vi "Tester 1.vi"() -> ()   [LabVIEW 2020]
doc: "211353135"
panel:
  in  "Numeric":i32
  # "Tester 1"
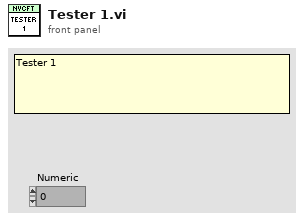
[diagram p1: front panel]
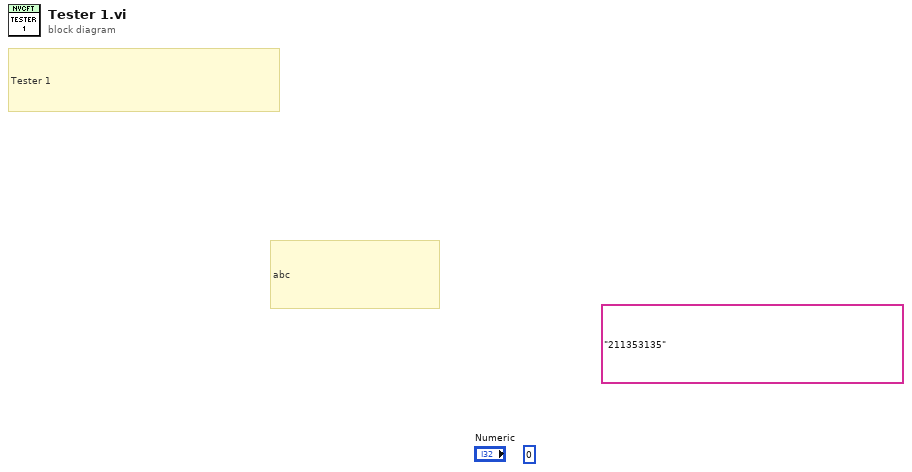
[diagram p0: block diagram]
diagram:
  (unwired) "211353135"
  (unwired) 0
  # "Tester 1"
  # "abc"
